vi "Send Text HMI.vi"() -> (1 "Chosen Text":string, 2 "Chosen Data Type":u16(ring) items=["Text File", "Image File", "Image", "Text"], 3 "Cancelled":bool)   [LabVIEW 2025]
panel:
  in  "Cancel":bool
  in  "Done":bool
  in  "String":string
  in  "Open File":bool
  in  "Enter Text":bool
  # "SEND TEXT"
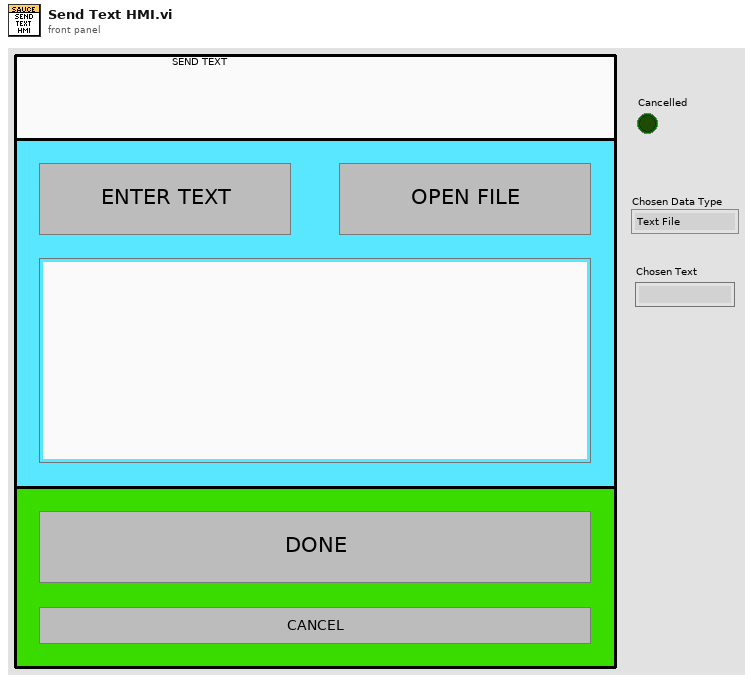
[diagram p1: front panel]
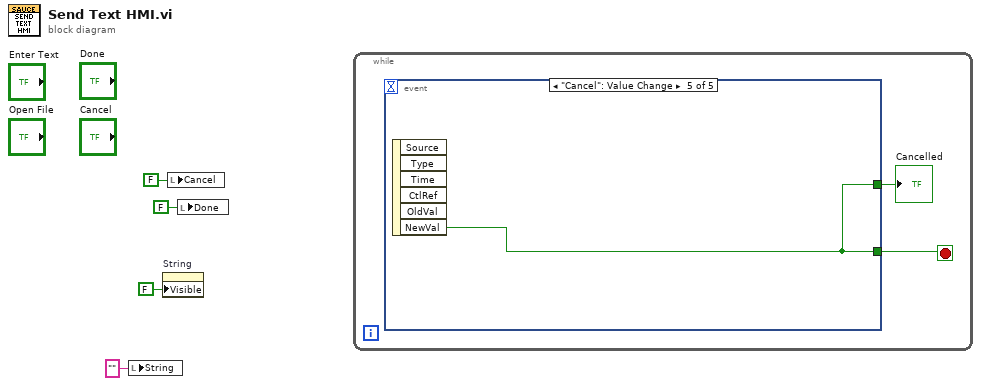
[diagram p0: block diagram]
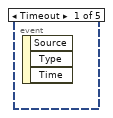
[diagram p2: hidden frame]
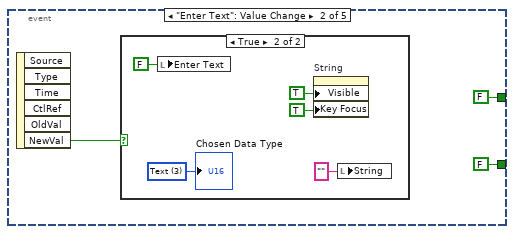
[diagram p3: hidden frame]
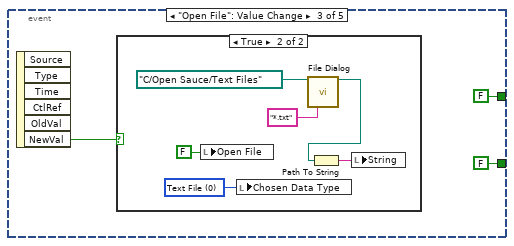
[diagram p5: hidden frame]
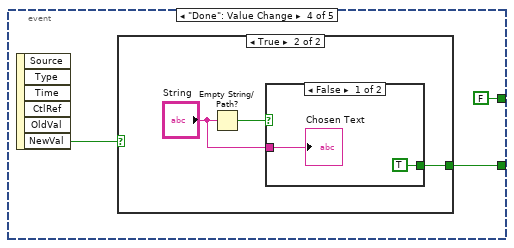
[diagram p7: hidden frame]
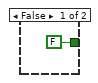
[diagram p8: hidden frame]
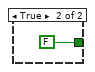
[diagram p9: hidden frame]
diagram:
  n1 = local write "String"("" ("String")) -> ()
  n2 = property on="String" class="Str"("Visible"=FALSE) -> ()  [unwired: 2 in, 2 out]
  n3 = local write "Cancel"(FALSE ("Cancel")) -> ()
  n4 = local write "Done"(FALSE ("Done")) -> ()
  n5 = while {
    stop <- w6 stop-if-true
    n6 = event shown="[4] \"Cancel\": Value Change" {
      selector: _ -> [_ _ _ _ _]
      dyn-events: _ -> [_ _ _ _ _]
      timeout: _ -> [_ _ _ _ _]
      tunnel: [_ FALSE FALSE w25 w34] -> w6
      tunnel: [_ FALSE FALSE FALSE w34] -> w5
      event Timeout {
        n7 = event-data() -> ()  [unwired: 1 in, 3 out]
      }
      event "Enter Text": Value Change {
        n8 = event-data() -> ("NewVal"=w9:bool)  [unwired: 1 in, 5 out]
        n9 = case shown="True" w9 {
          frame False {
          }
          frame True {
            w13 = u16 3 items=["Text File", "Image File", "Image", "Text"] ("Chosen Data Type")
            n10 = local write "Enter Text"(FALSE ("Enter Text")) -> ()
            n11 = property on="String" class="Str"("Visible"=TRUE, "Key Focus"=TRUE) -> ()  [unwired: 2 in, 2 out]
            n12 = local write "String"("" ("String")) -> ()
            "Chosen Data Type" <- w13
          }
        }
      }
      event "Open File": Value Change {
        n13 = event-data() -> ("NewVal"=w17:bool)  [unwired: 1 in, 5 out]
        n14 = case shown="True" w17 {
          frame False {
          }
          frame True {
            w21 = u16 0 items=["Text File", "Image File", "Image", "Text", ""] ("Chosen Data Type")
            n15 = local write "Open File"(FALSE ("Open File")) -> ()
            n16 = local write "Chosen Data Type"(w21) -> ()
            n17 = call "File Dialog"("start path"=path "C:/Open Sauce/Text Files", "pattern (all files)"="*.txt") -> ("selected path"=w19:path)  [unwired: 10 in, 3 out]
            n18 = Path To String(path=w19) -> (string=w20:string)
            n19 = local write "String"(w20) -> ()
          }
        }
      }
      event "Done": Value Change {
        n20 = event-data() -> ("NewVal"=w26:bool)  [unwired: 1 in, 5 out]
        n21 = case shown="True" w26 {
          tunnel: [FALSE w29] -> w25
          frame False {
          }
          frame True {
            n22 = Empty String/Path?(string/path="String") -> (empty?=w30:bool)
            n23 = case shown="False" w30 {
              tunnel: [TRUE FALSE] -> w29
              tunnel: "String" -> [w31 _]
              frame False {
                "Chosen Text" <- w31
              }
              frame True {
              }
            }
          }
        }
      }
      event "Cancel": Value Change {
        n24 = event-data() -> ("NewVal"=w34:bool)  [unwired: 1 in, 5 out]
      }
    }
    "Cancelled" <- w5
  }
